vi "Enter_LDA_Setup.vi"(0 "Show Panel":bool) -> ()   [LabVIEW 2010]
uses:
  Controls/BSA_info_Cluster.ctl
  BSA_Type.ctl
  Globals/Constants_global.vi
  Globals/LDA_meas_global_1.vi
  Globals/LDA_meas_global_2.vi
panel:
  in  "BSA Type":T1
  in  "BSA IP Number":string
  in  "Beam Alignment":u16(ring) items=["No Info", "Tunnel", "Model"]
  in  "45 Degree Mirror":bool
  in  "Swap BSA Order":bool
  in  "BSA Info":T2[](array[typedef]) {"Wavelength (nm)" format="%.1f"}
  in  "Probe Type":u16(ring) items=["14mm probe; Beam Separation=8mm; Focal Length=50mm", "14mm probe with beam expander; Beam Separation=16mm; Focal Length=120mm", "Test; Beam Separation=14mm; Focal Length=20mm", "Add Another LDA Probe"]
  in  "OK":bool
  # "BSA 1"
  # "BSA 2"
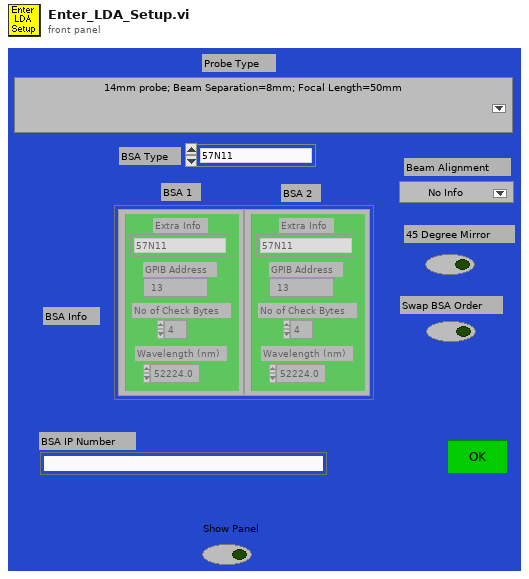
[diagram p1: front panel]
types:
  T1 = typedef "BSA_Type.ctl" = enum16{"57N11", "BSA F60"}
  T2 = typedef "BSA_info_Cluster.ctl" = cluster{"GPIB Address":string, "No of Check Bytes":i32, "Extra Info":string, "COLOUR":u32, "Wavelength (nm)":dbl}
  T3 = cluster{"Probe Name":string, "Beam Separation (mm)":dbl, "Focal Length (mm)":dbl}
  T4 = cluster{"Probe Name":string, "Beam Separation (mm)":dbl, "Focal Length (mm)":dbl}[]
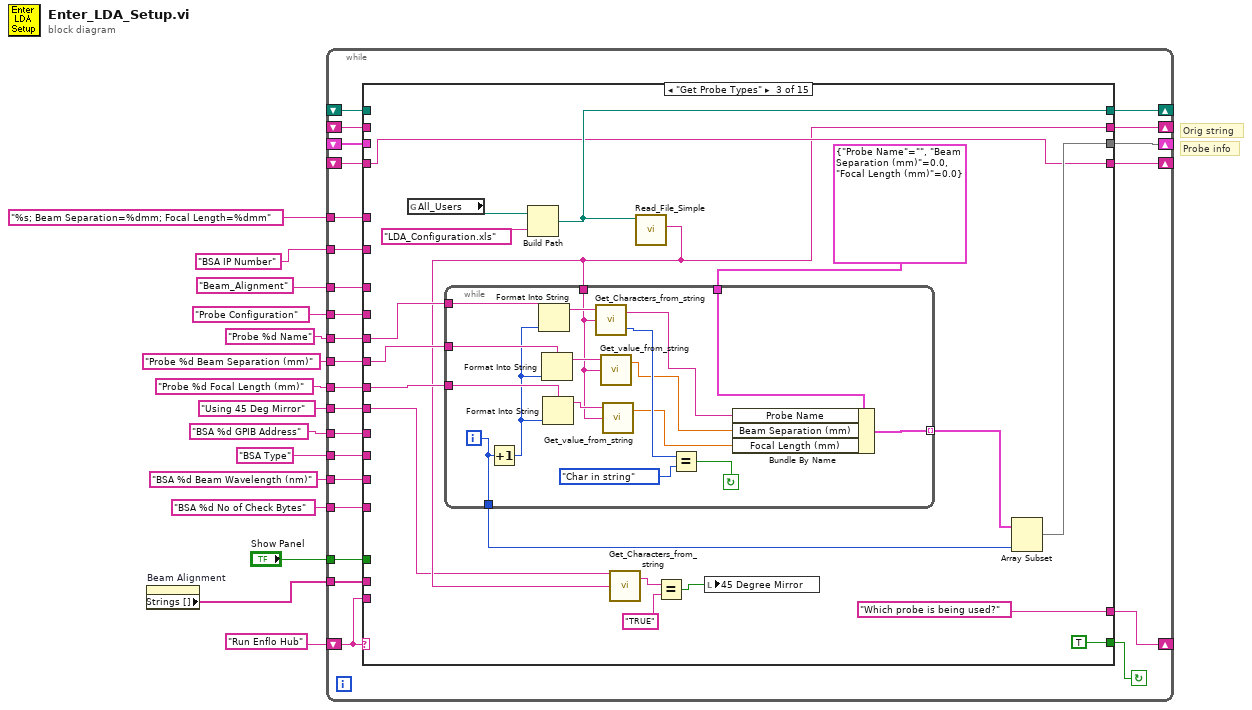
[diagram p0: block diagram]
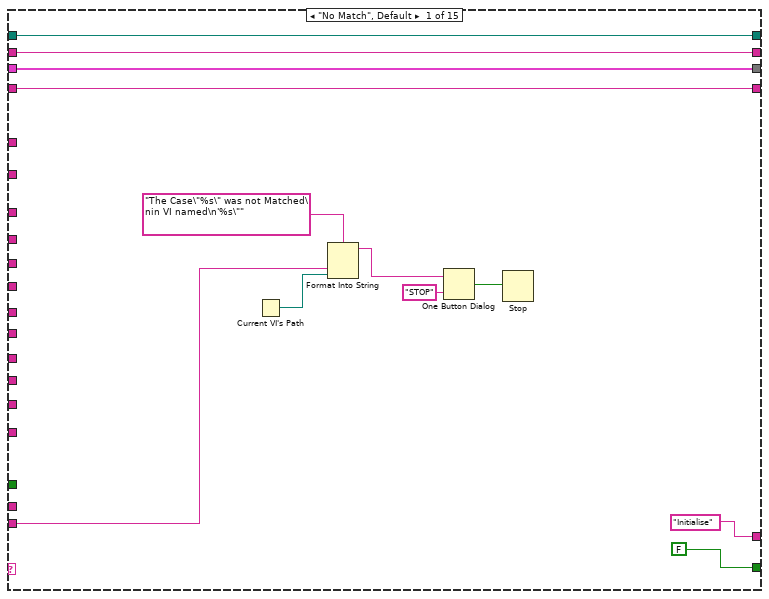
[diagram p2: hidden frame]
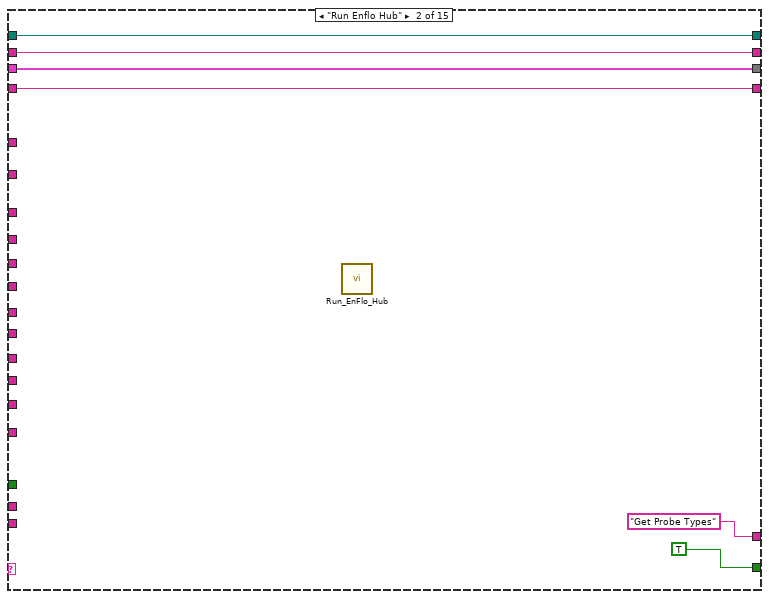
[diagram p3: hidden frame]
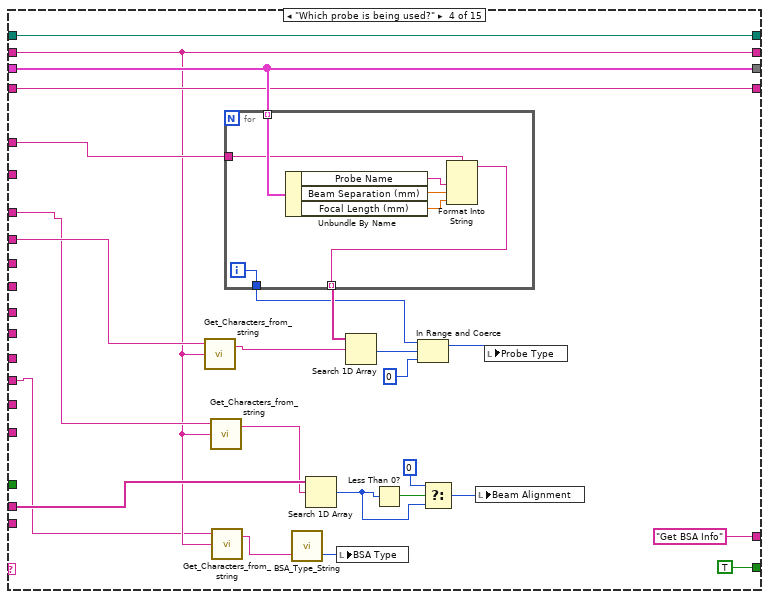
[diagram p4: hidden frame]
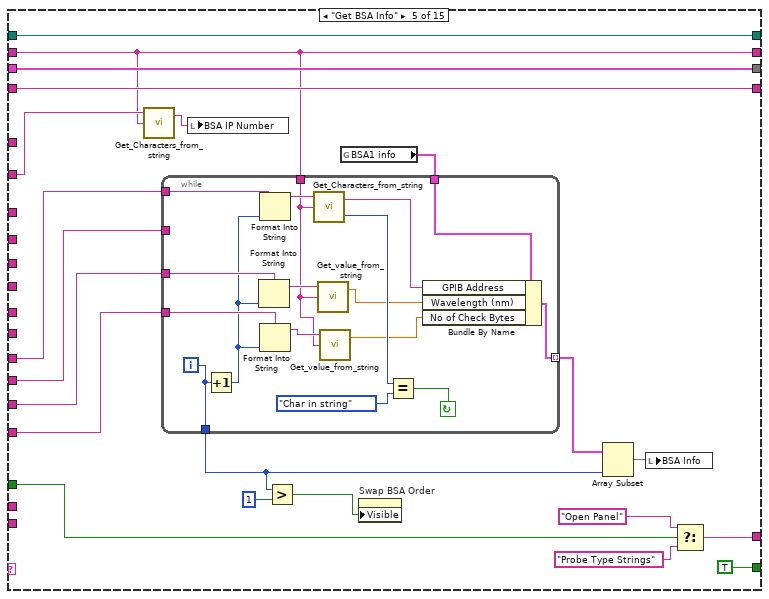
[diagram p5: hidden frame]
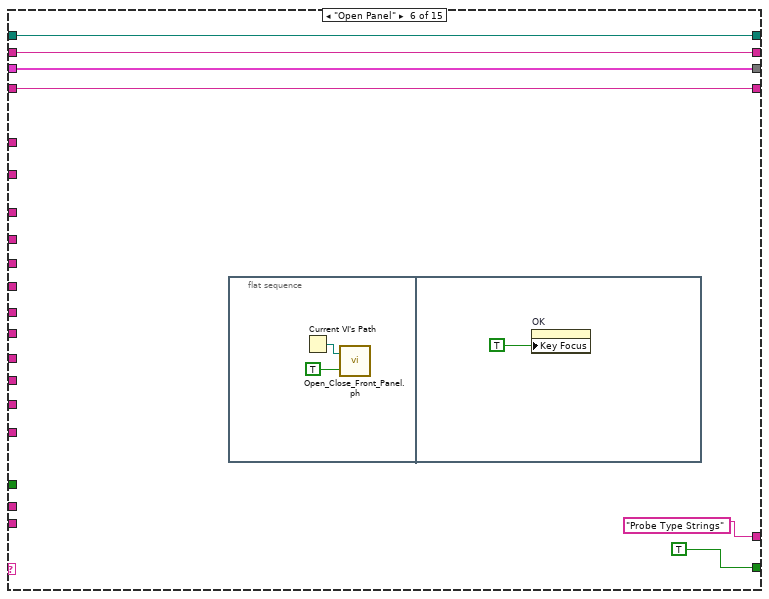
[diagram p6: hidden frame]
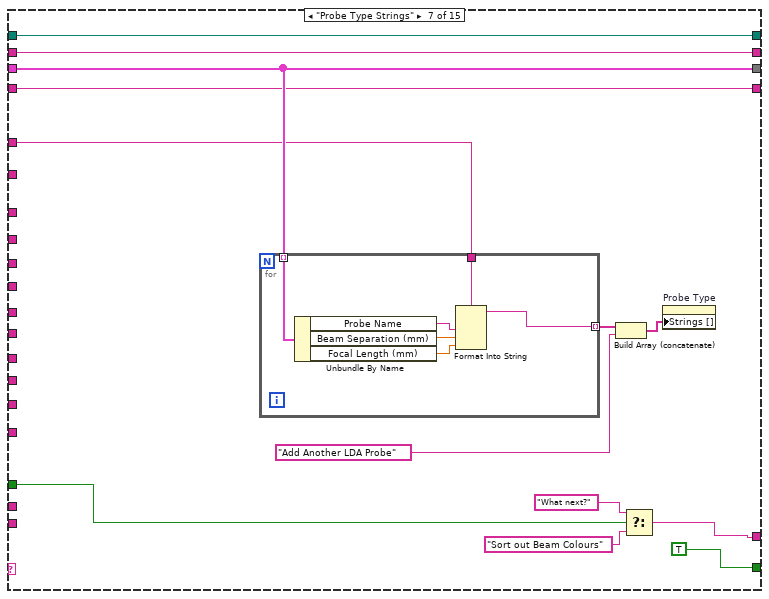
[diagram p7: hidden frame]
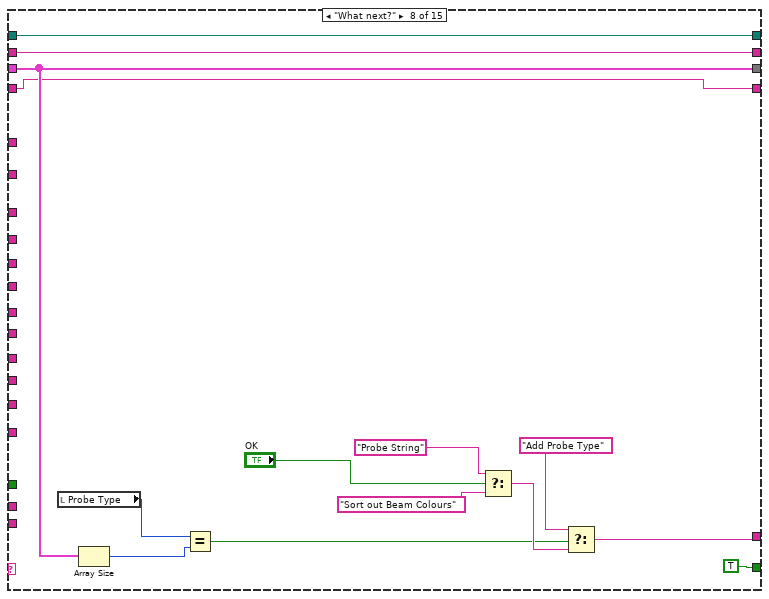
[diagram p8: hidden frame]
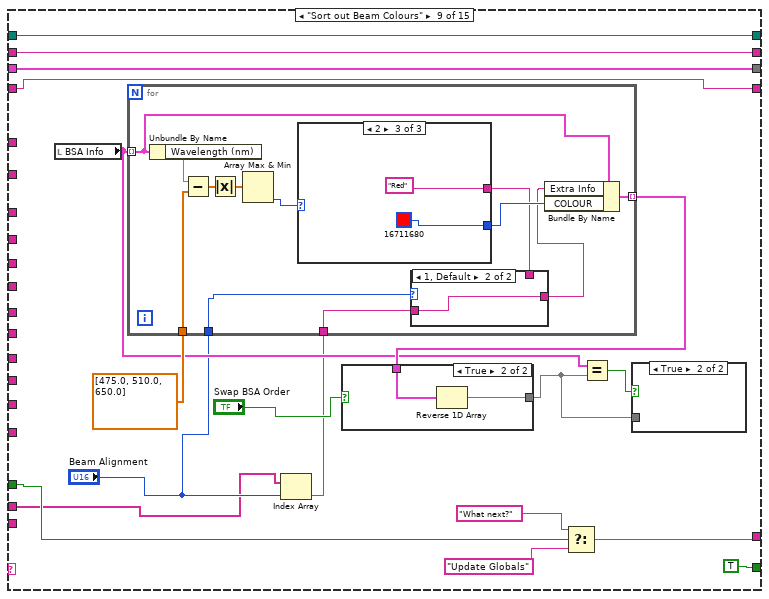
[diagram p9: hidden frame]
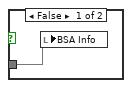
[diagram p10: hidden frame]
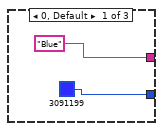
[diagram p13: hidden frame]
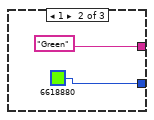
[diagram p14: hidden frame]
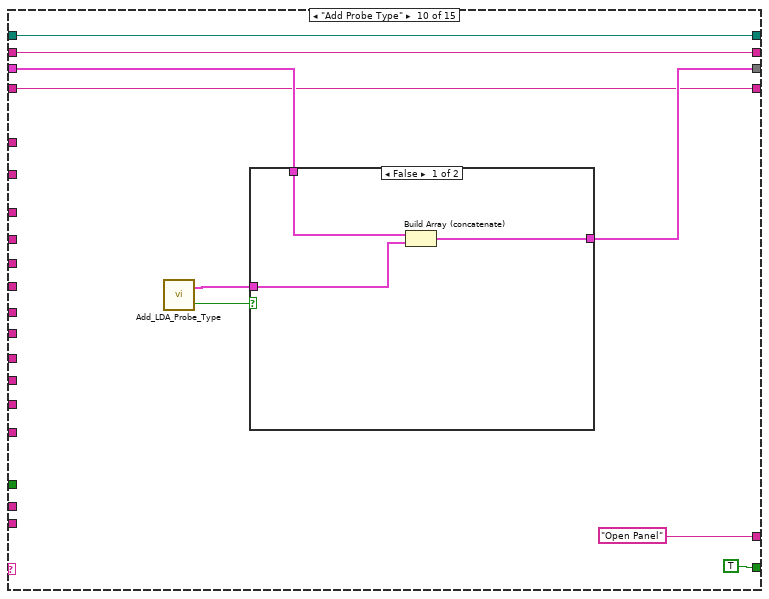
[diagram p15: hidden frame]
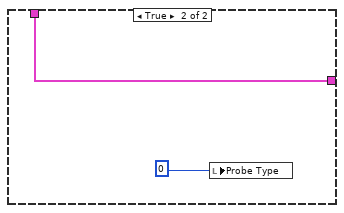
[diagram p16: hidden frame]
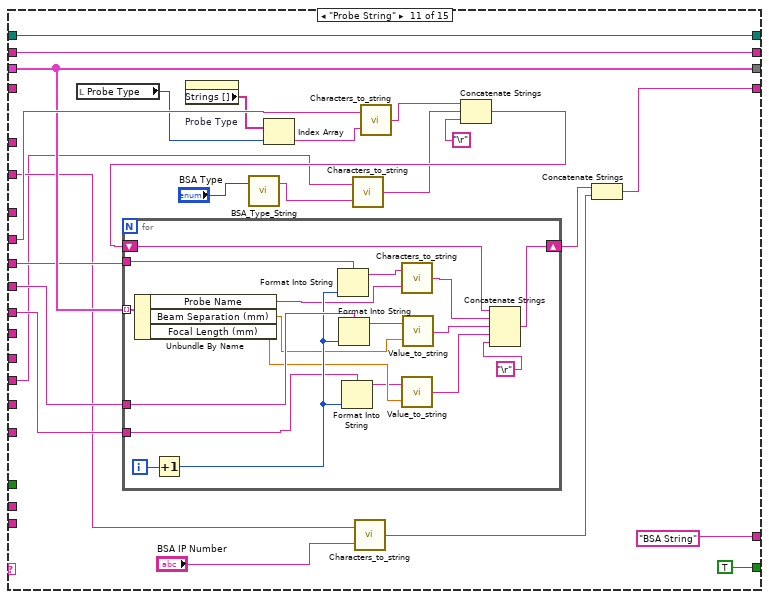
[diagram p17: hidden frame]
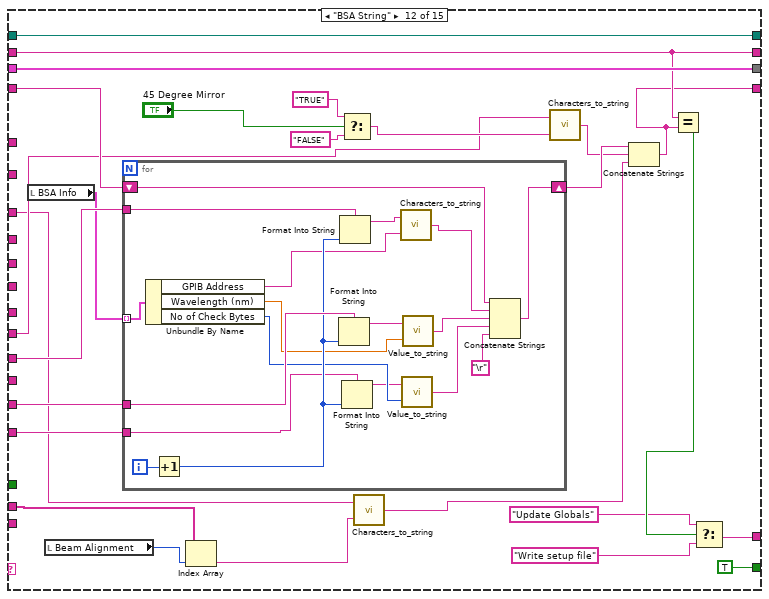
[diagram p18: hidden frame]
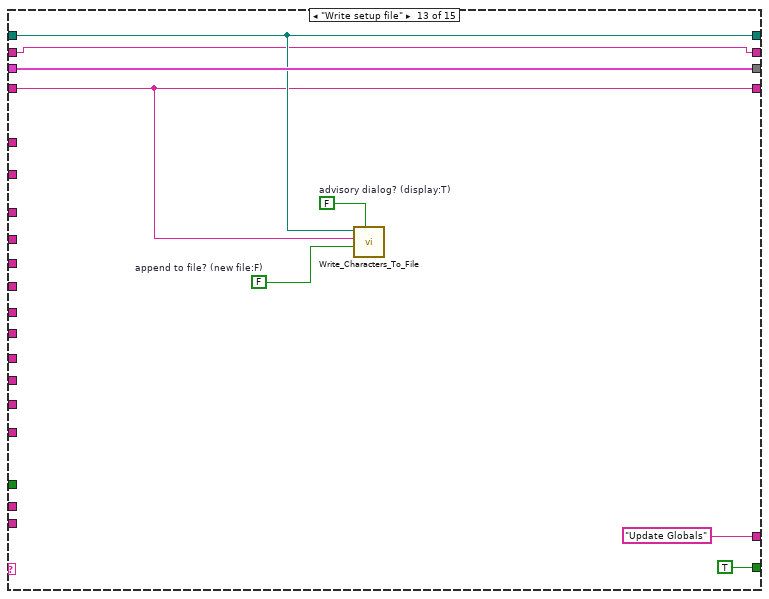
[diagram p19: hidden frame]
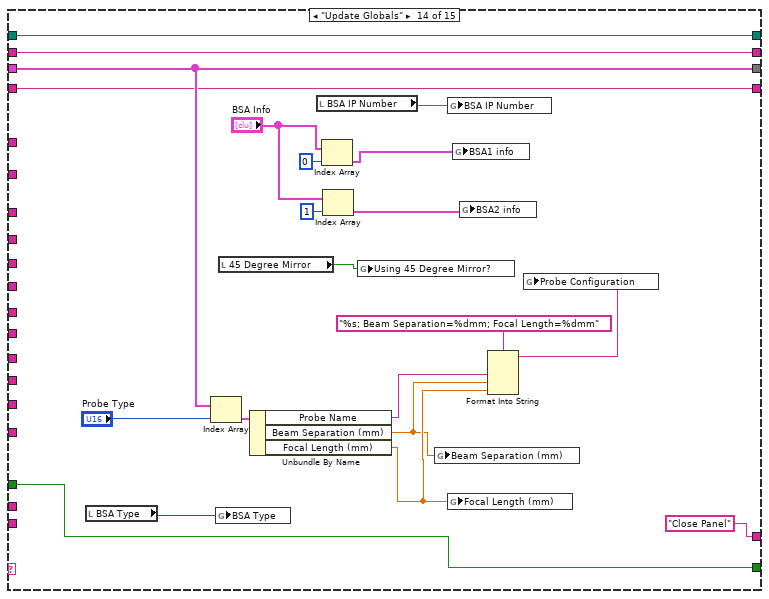
[diagram p20: hidden frame]
diagram:
  # "Orig string"
  # "Probe info"
  n1 = property on="Beam Alignment" class="Ring (strict)"() -> ("Strings []"=w3:string[])  [unwired: 2 in, 2 out]
  n2 = while {
    shift-left: "Run Enflo Hub" -> [w38]
    shift-right: [w39] -> _
    shift-right: [w37] -> _
    shift-left: _ -> [w36]
    tunnel: "Probe %d Name" -> [w35]
    shift-right: [w34] -> _
    shift-left: _ -> [w30]
    tunnel: "Probe %d Focal Length (mm)" -> [w33]
    tunnel: "Probe %d Beam Separation (mm)" -> [w32]
    shift-right: [w31] -> _
    shift-left: _ -> [w29]
    tunnel: "Probe Configuration" -> [w28]
    tunnel: "Show Panel" -> [w27]
    tunnel: "BSA %d GPIB Address" -> [w26]
    tunnel: "BSA Type" -> [w25]
    tunnel: "BSA %d Beam Wavelength (nm)" -> [w24]
    tunnel: "BSA %d No of Check Bytes" -> [w23]
    shift-right: [w21] -> _
    shift-left: _ -> [w22]
    tunnel: "%s; Beam Separation=%dmm; Focal Length=%dmm" ("format string") -> [w20]
    tunnel: "Using 45 Deg Mirror" -> [w19]
    tunnel: w3 -> [w18]
    tunnel: "Beam_Alignment" -> [w17]
    tunnel: "BSA IP Number" -> [w16]
    stop <- w40 continue-if-true
    n3 = case shown="\"Get Probe Types\"" w38 {
      tunnel: [FALSE TRUE TRUE TRUE TRUE TRUE TRUE TRUE TRUE TRUE TRUE TRUE TRUE w367 FALSE] -> w40
      tunnel: ["Initialise" "Get Probe Types" "Which probe is being used?" "Get BSA Info" w141 "Probe Type Strings" w173 w198 w217 "Open Panel" ("f") "BSA String" w316 "Update Globals" "Close Panel" "End"] -> w39
      tunnel: w38 -> [w47 _ _ _ _ _ _ _ _ _ _ _ _ _ _]
      tunnel: [w44 w56 w72 w114 w135 w166 w183 w202 w221 w254 w283 w324 w352 w375 w381] -> w37
      tunnel: w36 -> [w44 w56 _ w114 w135 w166 w183 w202 w221 w254 w283 w324 w352 w375 w381]
      tunnel: w35 -> [_ _ w73 _ _ _ _ _ _ _ w276 _ _ _ _]
      tunnel: [w43 w55 w63 w97 w126 w165 w182 w200 w220 w253 w278 w320 w351 w374 w378] -> w34
      tunnel: w33 -> [_ _ w71 _ _ _ _ _ _ _ w274 _ _ _ _]
      tunnel: w32 -> [_ _ w70 _ _ _ _ _ _ _ w275 _ _ _ _]
      tunnel: [w42 w54 w66 w113 w134 w164 w181 w196 w216 w248 w277 w323 w353 w370 w377] -> w31
      tunnel: w30 -> [w43 w55 _ w97 w126 w165 w182 w200 w220 w253 w278 w320 w351 w374 w378]
      tunnel: w29 -> [w42 w54 _ w113 w134 w164 w181 w196 w216 w249 w277 w323 w353 w370 w377]
      tunnel: w28 -> [_ _ _ w115 _ _ _ _ _ _ w282 _ _ _ _]
      tunnel: w27 -> [_ _ _ _ w143 _ w174 _ w210 _ _ _ _ w367 _]
      tunnel: w26 -> [_ _ _ _ w139 _ _ _ _ _ _ w327 _ _ _]
      tunnel: w25 -> [_ _ _ w96 w138 _ _ _ _ _ w262 _ _ _ _]
      tunnel: w24 -> [_ _ _ _ w137 _ _ _ _ _ _ w326 _ _ _]
      tunnel: w23 -> [_ _ _ _ w136 _ _ _ _ _ _ w325 _ _ _]
      tunnel: w22 -> [w41 w53 w64 w106 w128 w163 w180 w192 w215 w247 _ w321 w347 w363 w376]
      tunnel: [w41 w53 w64 w106 w128 w163 w180 w192 w215 w247 w267 w310 w347 w363 w376] -> w21
      tunnel: w20 -> [_ _ _ w105 _ _ w172 _ _ _ _ _ _ _ _]
      tunnel: w19 -> [_ _ w59 _ _ _ _ _ _ _ _ w308 _ _ _]
      tunnel: w18 -> [_ _ _ w103 _ _ _ _ w205 _ _ w305 _ _ _]
      tunnel: w17 -> [_ _ _ w104 _ _ _ _ _ _ _ w307 _ _ _]
      tunnel: w16 -> [_ _ _ _ w127 _ _ _ _ _ w269 _ _ _ _]
      frame "No Match", Default {
        n4 = Current VI's Path() -> (path=w46:path)
        n5 = Format Into String(format string="The Case\"%s\" was not Matched\nin VI named\n'%s\"" ("Format String"), w47, w46) -> (resulting string=w50:string)  [unwired: 2 in, 1 out]
        n6 = One Button Dialog(message=w50, button name ("OK")="STOP") -> (true=w48:bool)
        n7 = Stop(stop? (T)=w48) -> ()
      }
      frame "Run Enflo Hub" {
        n8 = call "Run_EnFlo_Hub.vi"() -> ()  [unwired: 8 out]
      }
      frame "Get Probe Types" {
        n9 = global read "Constants_global.vi" "All_Users"() -> (w75:path)
        n10 = Build Path(base path=w75, name or relative path="LDA_Configuration.xls") -> (appended path=w72:path)
        n11 = call "Read_File_Simple.vi"("Filename"=w72) -> ("string"=w63:string)  [unwired: 2 in, 7 out]
        n12 = while {
          tunnel: w73 -> [w93]
          tunnel: w63 -> [w87]
          tunnel: w71 -> [w91]
          tunnel: w70 -> [w90]
          tunnel: [w82] -> w69
          tunnel: T3 {"Probe Name"="", "Beam Separation (mm)"=0.0, "Focal Length (mm)"=0.0} -> [w81]
          tunnel: [w78] -> w67 mode=indexing
          i -> [w82]
          stop <- w83 continue-if-true
          n13 = Increment(x=w82) -> (x+1=w86:i32)
          n14 = Format Into String(format string=w93, w86) -> (resulting string=w92:string)  [unwired: 2 in, 1 out]
          n15 = Format Into String(format string=w90, w86) -> (resulting string=w89:string)  [unwired: 2 in, 1 out]
          n16 = Format Into String(format string=w91, w86) -> (resulting string=w88:string)  [unwired: 2 in, 1 out]
          n17 = call "Get_Characters_from_string.vi"("Input string"=w87, "Variable name"=w92) -> ("Status"=w84:enum16{"Char in string", "Char not in string"}, "Value"=w77:string)  [unwired: 1 in]
          n18 = call "Get_value_from_string.vi"("Input string"=w87, "Variable name"=w89) -> ("Value"=w79:dbl)  [unwired: 1 in, 1 out]
          n19 = call "Get_value_from_string.vi"("Input string"=w87, "Variable name"=w88) -> ("Value"=w80:dbl)  [unwired: 1 in, 1 out]
          n20 = Equal?(x=w84, y=enum16{"Char in string", "Char not in string"}."Char in string" ("Status")) -> (x = y?=w83:bool)
          n21 = Bundle By Name(cluster=w81, "Probe Name"=w77, "Beam Separation (mm)"=w79, "Focal Length (mm)"=w80) -> (w78:T3)
        }
        n22 = call "Get_Characters_from_string.vi"("Input string"=w63, "Variable name"=w59) -> ("Value"=w62:string)  [unwired: 1 in, 1 out]
        n23 = Equal?(x=w62, y="TRUE") -> (x = y?=w60:bool)
        n24 = local write "45 Degree Mirror"(w60) -> ()
        n25 = Array Subset(array=w67, length=w69) -> (w66:T4)  [unwired: 1 in]
      }
      frame "Which probe is being used?" {
        n26 = call "Get_Characters_from_string.vi"("Input string"=w97, "Variable name"=w115) -> ("Value"=w111:string)  [unwired: 1 in, 1 out]
        n27 = call "Get_Characters_from_string.vi"("Input string"=w97, "Variable name"=w104) -> ("Value"=w102:string)  [unwired: 1 in, 1 out]
        n28 = call "Get_Characters_from_string.vi"("Input string"=w97, "Variable name"=w96) -> ("Value"=w95:string)  [unwired: 1 in, 1 out]
        n29 = for {
          tunnel: w113 -> [w120] mode=indexing
          tunnel: [w118] -> w112 mode=indexing
          tunnel: [w124] -> w109
          tunnel: w105 -> [w119]
          i -> [w124]
          n30 = Unbundle By Name(w120) -> ("Probe Name"=w121:string, "Beam Separation (mm)"=w122:dbl, "Focal Length (mm)"=w123:dbl)
          n31 = Format Into String(format string=w119, w121, w122, w123) -> (resulting string=w118:string)  [unwired: 2 in, 1 out]
        }
        n32 = call "BSA_Type_String.vi"("BSA String in"=w95) -> ("BSA Type Out"=w94:T1)  [unwired: 1 in, 1 out]
        n33 = Search 1D Array(1D array=w103, element=w102) -> (index of element=w99:i32)  [unwired: 1 out]
        n34 = local write "BSA Type"(w94) -> ()
        n35 = Search 1D Array(1D array=w112, element=w111) -> (index of element=w110:i32)  [unwired: 1 out]
        n36 = Less Than 0?(x=w99) -> (x < 0?=w101:bool)
        n37 = In Range and Coerce(upper limit=w109, x=w110, lower limit=0) -> (coerced(x)=w107:i32)  [unwired: 1 out]
        n38 = Select(t=0, s=w101, f=w99) -> (s? t:f=w98:i32)
        n39 = local write "Beam Alignment"(w98) -> ()
        n40 = local write "Probe Type"(w107) -> ()
      }
      frame "Get BSA Info" {
        n41 = call "Get_Characters_from_string.vi"("Input string"=w126, "Variable name"=w127) -> ("Value"=w125:string)  [unwired: 1 in, 1 out]
        n42 = local write "BSA IP Number"(w125) -> ()
        n43 = global read "LDA_meas_global_1.vi" "BSA1 info"() -> (w140:T2)
        n44 = while {
          tunnel: w138 -> [_]
          tunnel: w126 -> [w146]
          tunnel: w136 -> [w162]
          tunnel: w137 -> [w161]
          tunnel: [w156] -> w131
          tunnel: w140 -> [w155]
          tunnel: [w154] -> w144 mode=indexing
          tunnel: w139 -> [w151]
          i -> [w156]
          stop <- w157 continue-if-true
          n45 = Increment(x=w156) -> (x+1=w152:i32)
          n46 = Format Into String(format string=w161, w152) -> (resulting string=w160:string)  [unwired: 2 in, 1 out]
          n47 = Format Into String(format string=w151, w152) -> (resulting string=w153:string)  [unwired: 2 in, 1 out]
          n48 = Format Into String(format string=w162, w152) -> (resulting string=w159:string)  [unwired: 2 in, 1 out]
          n49 = call "Get_Characters_from_string.vi"("Input string"=w146, "Variable name"=w153) -> ("Status"=w150:enum16{"Char in string", "Char not in string"}, "Value"=w149:string)  [unwired: 1 in]
          n50 = call "Get_value_from_string.vi"("Input string"=w146, "Variable name"=w160) -> ("Value"=w148:dbl)  [unwired: 1 in, 1 out]
          n51 = call "Get_value_from_string.vi"("Input string"=w146, "Variable name"=w159) -> ("Value"=w147:dbl)  [unwired: 1 in, 1 out]
          n52 = Equal?(x=w150, y=enum16{"Char in string", "Char not in string"}."Char in string" ("Status")) -> (x = y?=w157:bool)
          n53 = Bundle By Name(cluster=w155, "GPIB Address"=w149, "Wavelength (nm)"=w148, "No of Check Bytes"=w147) -> (w154:T2)
        }
        n54 = Greater?(x=w131, y=1) -> (0:w129:bool)
        n55 = property on="Swap BSA Order" class="Bool"("Visible"=w129) -> ()  [unwired: 2 in, 2 out]
        n56 = Array Subset(array=w144, length=w131) -> (w133:T2[])  [unwired: 1 in]
        n57 = local write "BSA Info"(w133) -> ()
        n58 = Select(t="Open Panel", s=w143, f="Probe Type Strings") -> (s? t:f=w141:string)
      }
      frame "Open Panel" {
        n59 = flat-sequence {
          frame #0 {
            n60 = Current VI's Path() -> (path=w170:path)
            n61 = call "Open_Close_Front_Panel.ph.vi"("Front Panel Window:Open"=TRUE, "VI path"=w170) -> ()  [unwired: 2 out]
          }
          frame #1 {
            n62 = property on="OK" class="Bool"("Key Focus"=TRUE) -> ()  [unwired: 2 in, 2 out]
          }
        }
      }
      frame "Probe Type Strings" {
        n63 = for {
          tunnel: w181 -> [w190] mode=indexing
          tunnel: [w189] -> w179 mode=indexing
          tunnel: w172 -> [w185]
          n64 = Unbundle By Name(w190) -> ("Probe Name"=w188:string, "Beam Separation (mm)"=w187:dbl, "Focal Length (mm)"=w186:dbl)
          n65 = Format Into String(format string=w185, w188, w187, w186) -> (resulting string=w189:string)  [unwired: 2 in, 1 out]
        }
        n66 = Build Array (concatenate)(w179, "Add Another LDA Probe" ("Probe Name")) -> (w178:string[])
        n67 = Select(t="What next?", s=w174, f="Sort out Beam Colours") -> (s? t:f=w173:string)
        n68 = property on="Probe Type" class="Ring (strict)"("Strings []"=w178) -> ()  [unwired: 2 in, 2 out]
      }
      frame "What next?" {
        n69 = local read "Probe Type"() -> (w194:u16)
        n70 = Array Size(array=w196) -> (size(s)=w195:i32)
        n71 = Equal?(x=w194, y=w195) -> (x = y?=w193:bool)
        n72 = Select(t="Probe String", s="OK", f="Sort out Beam Colours") -> (s? t:f=w199:string)
        n73 = Select(t="Add Probe Type", s=w193, f=w199) -> (s? t:f=w198:string)
      }
      frame "Sort out Beam Colours" {
        n74 = local read "BSA Info"() -> (w214:T2[])
        n75 = Index Array(array=w205, index="Beam Alignment") -> (element=w206:string)
        n76 = for {
          tunnel: w214 -> [w233] mode=indexing
          tunnel: dbl[] [475.0, 510.0, 650.0] -> [w237]
          tunnel: [w231] -> w218 mode=indexing
          tunnel: "Beam Alignment" -> [w230]
          tunnel: w206 -> [w227]
          n77 = Unbundle By Name(w233) -> ("Wavelength (nm)"=w238:dbl)
          n78 = Subtract(x=w238, y=w237) -> (x-y=w236:dbl[])
          n79 = Absolute Value(x=w236) -> (abs(x)=w235:dbl[])
          n80 = Array Max & Min(array=w235) -> (min index (indices)=w234:i32)  [unwired: 3 out]
          n81 = case shown="2" w234 {
            tunnel: ["Blue" "Green" "Red"] -> w228
            tunnel: [u32 3091199 u32 6618880 u32 16711680] -> w232
            frame 0, Default {
            }
            frame 1 {
            }
            frame 2 {
            }
          }
          n82 = case shown="1, Default" w230 {
            tunnel: [w239 w240] -> w229
            tunnel: w228 -> [w239 _]
            tunnel: w227 -> [_ w240]
            frame 0 {
            }
            frame 1, Default {
            }
          }
          n83 = Bundle By Name(cluster=w233, "Extra Info"=w229, "COLOUR"=w232) -> (w231:T2)
        }
        n84 = case shown="True" "Swap BSA Order" {
          tunnel: w218 -> [w224 w226]
          tunnel: [w224 w225] -> w212
          frame False {
          }
          frame True {
            n85 = Reverse 1D Array(array=w226) -> (reversed array=w225:T2[])
          }
        }
        n86 = Select(t="What next?" ("f"), s=w210, f="Update Globals") -> (s? t:f=w217:string)
        n87 = Equal?(x=w214, y=w212) -> (x = y?=w213:bool)
        n88 = case shown="True" w213 {
          tunnel: w212 -> [w223 _]
          frame False {
            n89 = local write "BSA Info"(w223) -> ()
          }
          frame True {
          }
        }
      }
      frame "Add Probe Type" {
        n90 = call "Add_LDA_Probe_Type.vi"() -> ("Cancel Out"=w251:bool, "New LDA Probe Type Out"=w250:T3)  [unwired: 3 out]
        n91 = case shown="False" w251 {
          tunnel: w250 -> [w258 _]
          tunnel: w249 -> [w257 w260]
          tunnel: [w256 w260] -> w248
          frame False {
            n92 = Build Array (concatenate)(w257, w258) -> (w256:T4)
          }
          frame True {
            n93 = local write "Probe Type"(0) -> ()
          }
        }
      }
      frame "Probe String" {
        n94 = local read "Probe Type"() -> (w271:u16)
        n95 = property on="Probe Type" class="Ring (strict)"() -> ("Strings []"=w272:string[])  [unwired: 2 in, 2 out]
        n96 = call "BSA_Type_String.vi"("BSA Type"="BSA Type") -> ("BSA String Out"=w263:string)  [unwired: 1 in, 1 out]
        n97 = Index Array(array=w272, index=w271) -> (element=w270:string)
        n98 = call "Characters_to_string.vi"("Characters to write"=w263, "Label for characters"=w262) -> ("Output string"=w261:string)
        n99 = call "Characters_to_string.vi"("Characters to write"="BSA IP Number", "Label for characters"=w269) -> ("Output string"=w266:string)
        n100 = call "Characters_to_string.vi"("Characters to write"=w270, "Label for characters"=w282) -> ("Output string"=w281:string)
        n101 = Concatenate Strings(w281, w261, "\r") -> (w279:string)
        n102 = for {
          tunnel: w276 -> [w301]
          tunnel: w275 -> [w300]
          tunnel: w274 -> [w298]
          shift-right: [w294] -> w268
          shift-left: w279 -> [w286]
          tunnel: w277 -> [w287] mode=indexing
          i -> [w302]
          n103 = Unbundle By Name(w287) -> ("Probe Name"=w293:string, "Beam Separation (mm)"=w292:dbl, "Focal Length (mm)"=w291:dbl)
          n104 = Increment(x=w302) -> (x+1=w299:i32)
          n105 = Format Into String(format string=w301, w299) -> (resulting string=w288:string)  [unwired: 2 in, 1 out]
          n106 = Format Into String(format string=w300, w299) -> (resulting string=w289:string)  [unwired: 2 in, 1 out]
          n107 = Format Into String(format string=w298, w299) -> (resulting string=w290:string)  [unwired: 2 in, 1 out]
          n108 = call "Characters_to_string.vi"("Characters to write"=w293, "Label for characters"=w288) -> ("Output string"=w295:string)
          n109 = call "Value_to_string.vi"("Value"=w291, "Label for value"=w290) -> ("Output string"=w297:string)  [unwired: 1 in]
          n110 = call "Value_to_string.vi"("Value"=w292, "Label for value"=w289) -> ("Output string"=w296:string)  [unwired: 1 in]
          n111 = Concatenate Strings(w286, w295, w296, w297, "\r") -> (w294:string)
        }
        n112 = Concatenate Strings(w268, w266) -> (w267:string)
      }
      frame "BSA String" {
        n113 = local read "BSA Info"() -> (w322:T2[])
        n114 = local read "Beam Alignment"() -> (w306:u16)
        n115 = for {
          tunnel: w327 -> [w345]
          tunnel: w326 -> [w344]
          tunnel: w325 -> [w342]
          shift-right: [w337] -> w311
          shift-left: w321 -> [w330]
          tunnel: w322 -> [w341] mode=indexing
          i -> [w346]
          n116 = Unbundle By Name(w341) -> ("GPIB Address"=w335:string, "Wavelength (nm)"=w334:dbl, "No of Check Bytes"=w333:i32)
          n117 = Increment(x=w346) -> (x+1=w343:i32)
          n118 = Format Into String(format string=w344, w343) -> (resulting string=w331:string)  [unwired: 2 in, 1 out]
          n119 = Format Into String(format string=w345, w343) -> (resulting string=w336:string)  [unwired: 2 in, 1 out]
          n120 = Format Into String(format string=w342, w343) -> (resulting string=w332:string)  [unwired: 2 in, 1 out]
          n121 = call "Characters_to_string.vi"("Characters to write"=w335, "Label for characters"=w336) -> ("Output string"=w338:string)
          n122 = call "Value_to_string.vi"("Value"=w333, "Label for value"=w332) -> ("Output string"=w340:string)  [unwired: 1 in]
          n123 = call "Value_to_string.vi"("Value"=w334, "Label for value"=w331) -> ("Output string"=w339:string)  [unwired: 1 in]
          n124 = Concatenate Strings(w330, w338, w339, w340, "\r") -> (w337:string)
        }
        n125 = Index Array(array=w305, index=w306) -> (element=w304:string)
        n126 = Select(t="TRUE", s="45 Degree Mirror", f="FALSE") -> (s? t:f=w312:string)
        n127 = call "Characters_to_string.vi"("Characters to write"=w304, "Label for characters"=w307) -> ("Output string"=w303:string)
        n128 = call "Characters_to_string.vi"("Characters to write"=w312, "Label for characters"=w308) -> ("Output string"=w309:string)
        n129 = Concatenate Strings(w311, w309, w303) -> (w310:string)
        n130 = Equal?(x=w320, y=w310) -> (x = y?=w319:bool)
        n131 = Select(t="Update Globals", s=w319, f="Write setup file") -> (s? t:f=w316:string)
      }
      frame "Write setup file" {
        w349 = FALSE  # append to file? (new file:F)
        w350 = FALSE  # advisory dialog? (display:T)
        n132 = call "Write_Characters_To_File.vi"("file path (dialog if empty)"=w352, "advisory dialog? (display:T)"=w350, "character string"=w347, "append to file? (new file:F)"=w349) -> ()  [unwired: 1 in, 4 out]
      }
      frame "Update Globals" {
        n133 = local read "BSA Type"() -> (w355:T1)
        n134 = Index Array(array=w370, index="Probe Type") -> (element=w371:T3)
        n135 = global write "LDA_meas_global_1.vi" "BSA Type"(w355) -> ()
        n136 = local read "45 Degree Mirror"() -> (w357:bool)
        n137 = Unbundle By Name(w371) -> ("Probe Name"=w359:string, "Beam Separation (mm)"=w360:dbl, "Focal Length (mm)"=w361:dbl)
        n138 = local read "BSA IP Number"() -> (w356:string)
        n139 = Index Array(array="BSA Info", index=0) -> (element=w365:T2)
        n140 = Index Array(array="BSA Info", index=1) -> (element=w364:T2)
        n141 = global write "LDA_meas_global_1.vi" "Using 45 Degree Mirror?"(w357) -> ()
        n142 = global write "LDA_meas_global_1.vi" "Beam Separation (mm)"(w360) -> ()
        n143 = global write "LDA_meas_global_1.vi" "BSA IP Number"(w356) -> ()
        n144 = global write "LDA_meas_global_1.vi" "Focal Length (mm)"(w361) -> ()
        n145 = global write "LDA_meas_global_1.vi" "BSA1 info"(w365) -> ()
        n146 = global write "LDA_meas_global_2.vi" "BSA2 info"(w364) -> ()
        n147 = Format Into String(format string="%s; Beam Separation=%dmm; Focal Length=%dmm", w359, w360, w361) -> (resulting string=w358:string)  [unwired: 2 in, 1 out]
        n148 = global write "LDA_meas_global_1.vi" "Probe Configuration"(w358) -> ()
      }
      frame "Close Panel" {
        n149 = Current VI's Path() -> (path=w380:path)
        n150 = call "Open_Close_Front_Panel.ph.vi"("Front Panel Window:Open"=FALSE, "VI path"=w380) -> ()  [unwired: 2 out]
      }
    }
  }
